vi "Wrap Sequence File.vi"(8 "error in (no error)":errorcluster, 10 "TS SequenceFile":refnum<k7>, 11 "Engine in":refnum<class "Engine.lvclass">) -> (0 "error out":errorcluster, 2 "TSnax:SequenceFile":refnum<class "SequenceFile.lvclass">, 3 "Engine out":refnum<class "Engine.lvclass">)   [LabVIEW 2020, in "TSnax.lvlib" / "Engine.lvclass"]
uses:
  Engine.lvclass
  Engine.lvclass/Engine.ctl
  SequenceFile/SequenceFile.lvclass
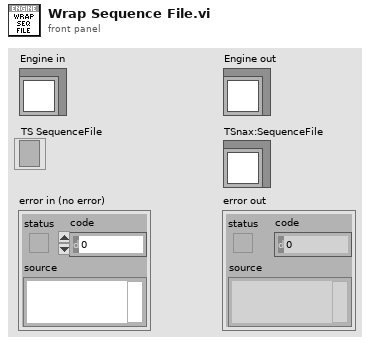
[diagram p1: front panel]
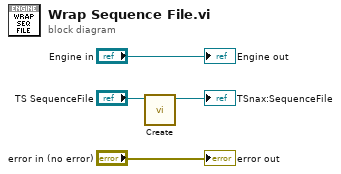
[diagram p0: block diagram]
diagram:
  n1 = call "Create.vi"("SequenceFile"="TS SequenceFile") -> ("SequenceFile out"=→"TSnax:SequenceFile":refnum<class "SequenceFile.lvclass">)  [unwired: 9 in, 1 out]
  "error out" <- "error in (no error)"
  "Engine out" <- "Engine in"
